vi "StellarNet Initialize All Spectrometers, ext precision.vi"(7 "Path of swdll.dll":path=path "C:/program files/StellarNet/SpectraWiz/swdll.dll", 8 "error in":errorcluster, 9 "Spectrometer Coefficients file":path=path "StellarNet LV-SpectraWiz-1ch Spectrometer Coefficients, ext precision.xml", 10 "Location of SpectraWiz":path=path "C:/program files/StellarNet/SpectraWiz", 11 "Name of SpectraWiz initialization file":path=path "sw.ini") -> (0 "error out":errorcluster, 1 "Auto-load":bool[](array[boolean])=[TRUE], 2 "Multi Channel Coeffs & WLs":T1(array[cluster])=[{"Coefficients"=[0.0, 0.0001294, 315.66, 0.0], "Wavelengths"=array[2051 elements]}], 3 "Number of Channels":i32=1, 5 "Detector Types":u16[](array[numeric]))   [LabVIEW 2023]
uses:
  StellarNet Get-Set Channel Coefficients, ext precision.vi
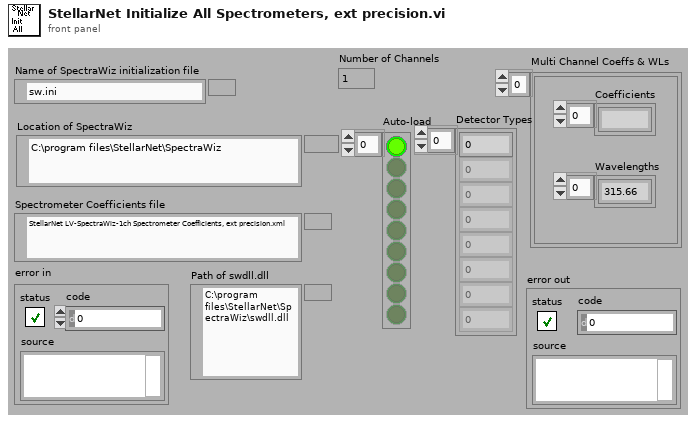
[diagram p1: front panel]
types:
  T1 = cluster{"Coefficients":ext[], "Wavelengths":dbl[]}[]
  T2 = cluster{"Coefficients":ext[], "Coefficients":dbl[]}
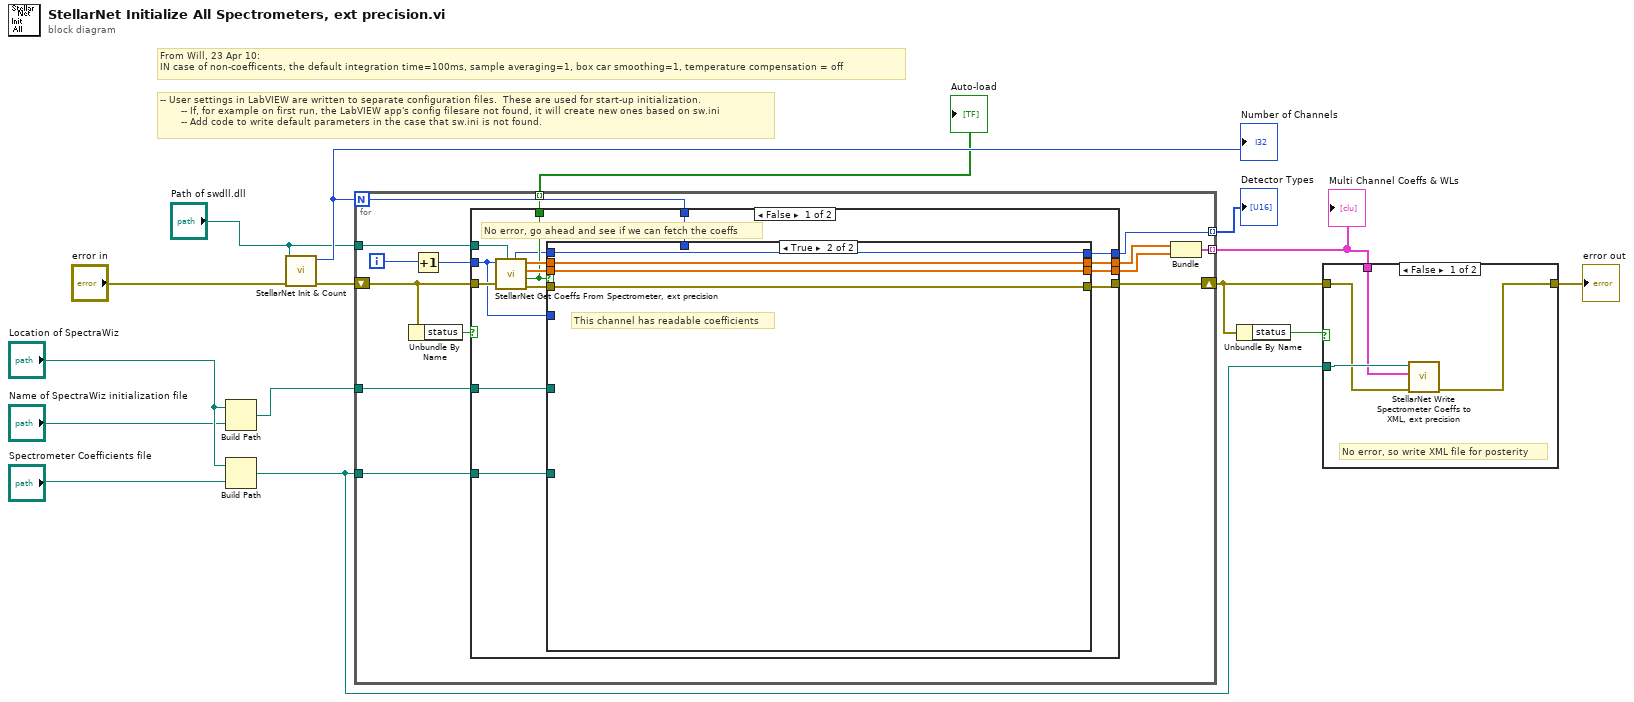
[diagram p0: block diagram]
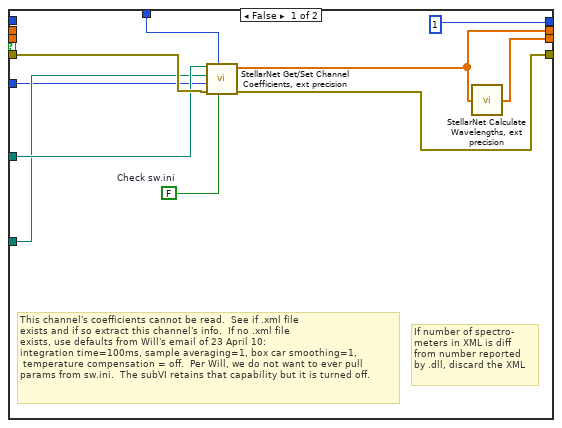
[diagram p3: hidden frame]
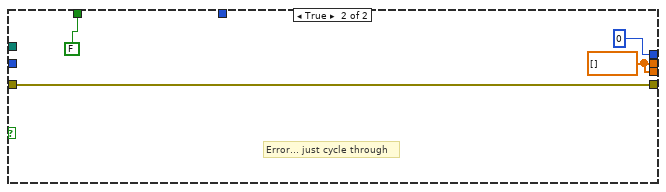
[diagram p4: hidden frame]
diagram:
  # "-- User settings in LabVIEW are written to separate configuration files.  These are used for start-up initialization.\n       -- If, for example on first run, the LabVIEW app's config filesare not found, it will create new ones based on sw.ini\n       -- Add code to write default parameters in the case that sw.ini is not found."
  # "From Will, 23 Apr 10:\nIN case of non-coefficents, the default integration time=100ms, sample averaging=1, box car smoothing=1, temperature compensation = off"
  n1 = Build Path(base path="Location of SpectraWiz", name or relative path="Name of SpectraWiz initialization file") -> (appended path=w11:path)
  n2 = Build Path(base path="Location of SpectraWiz", name or relative path="Spectrometer Coefficients file") -> (appended path=w7:path)
  n3 = call "StellarNet Init & Count.vi"("error in (no error)"="error in", "reference"="Path of swdll.dll") -> ("error out"=w13:errorcluster, "Number of Channels"=w14:i32)  [unwired: 8 in]
  "Number of Channels" <- w14
  n4 = for {
    N: w14 -> [w19]
    shift-right: [w26] -> w9
    shift-left: w13 -> [w28]
    tunnel: [w23] -> w6 mode=indexing
    tunnel: w7 -> [w22]
    tunnel: w11 -> [w21]
    tunnel: [w18] -> w3 mode=indexing
    tunnel: [w17] -> w2 mode=indexing
    tunnel: "Path of swdll.dll" -> [w16]
    i -> [w20]
    n5 = Unbundle By Name(w28) -> ("status"=w29:bool)
    n6 = Increment(x=w20) -> (x+1=w27:i32)
    n7 = case shown="False" w29 {
      tunnel: w28 -> [w44 w62]
      tunnel: w27 -> [w34 _]
      tunnel: [w38 w62] -> w26
      tunnel: [w41 w61] -> w25
      tunnel: [w40 w61] -> w24
      tunnel: w22 -> [w37 _]
      tunnel: w21 -> [w36 _]
      tunnel: w19 -> [w35 _]
      tunnel: [w33 FALSE ("Valid")] -> w18
      tunnel: [w31 u16 0 ("M (detector specifier)")] -> w17
      tunnel: w16 -> [w30 _]
      frame False {
        # "No error, go ahead and see if we can fetch the coeffs"
        n8 = call "StellarNet Get Coeffs From Spectrometer, ext precision.vi"("Path of sw.dll"=w30, "error in"=w44, "Channel\n(1-based)"=w34) -> ("error out"=w39:errorcluster, "Valid"=w33:bool, "Wavelengths"=w42:dbl[], "Coefficients"=w43:ext[], "M (detector specifier)"=w32:u16)  [unwired: 4 in]
        n9 = case shown="True" w33 {
          tunnel: w43 -> [_ w58]
          tunnel: w42 -> [_ w57]
          tunnel: [w53 w58] -> w41
          tunnel: [w54 w57] -> w40
          tunnel: w39 -> [w52 w56]
          tunnel: [w51 w56] -> w38
          tunnel: w37 -> [w49 _]
          tunnel: w36 -> [w50 _]
          tunnel: w35 -> [w47 _]
          tunnel: w34 -> [w48 _]
          tunnel: w32 -> [_ w55]
          tunnel: [u16 1 ("M (detector specifier)") w55] -> w31
          frame False {
            w46 = FALSE  # Check sw.ini
            # "If number of spectro-\nmeters in XML is diff\nfrom number reported\nby .dll, discard the XML"
            # "This channel's coefficients cannot be read.  See if .xml file \nexists and if so extract this channel's info.  If no .xml file \nexists, use defaults from Will's email of 23 April 10:\nintegration time=100ms, sample averaging=1, box car smoothing=1,\n temperature compensation = off.  Per Will, we do not want to ever pull\nparams from sw.ini.  The subVI retains that capability but it is turned off."
            n10 = call "StellarNet Get/Set Channel Coefficients, ext precision.vi"("Check sw.ini"=w46, "Number of Channels (from .dll)"=w47, "error in (no error)"=w52, "Channel (1-based)"=w48, "Location of Spectrometer Coefficients xml file"=w49, "Location of SpectraWiz ini file"=w50) -> ("error out"=w51:errorcluster, "Coefficients"=w53:ext[])  [unwired: 4 in]
            n11 = call "StellarNet Calculate Wavelengths, ext precision.vi"("C's"=w53) -> ("Wavelengths"=w54:dbl[])
          }
          frame True {
            # "This channel has readable coefficients"
          }
        }
      }
      frame True {
        w61 = dbl[] [] ("Coefficients")
        # "Error... just cycle through"
      }
    }
    n12 = Bundle("Coefficients"=w25, "Coefficients"=w24) -> (w23:T2)  [unwired: 1 in]
  }
  "Multi Channel Coeffs & WLs" <- w6
  "Auto-load" <- w3
  "Detector Types" <- w2
  n13 = Unbundle By Name(w9) -> ("status"=w10:bool)
  n14 = case shown="False" w10 {
    tunnel: w9 -> [w64 w67]
    tunnel: [w63 w67] -> w8
    tunnel: w7 -> [w66 _]
    tunnel: w6 -> [w65 _]
    frame False {
      # "No error, so write XML file for posterity"
      n15 = call "StellarNet Write Spectrometer Coeffs to XML, ext precision.vi"("error in (no error)"=w64, "Multi Channel Coefficients & WLs"=w65, "XML File Path"=w66) -> ("error out"=w63:errorcluster)  [unwired: 8 in]
    }
    frame True {
    }
  }
  "error out" <- w8
